vi "Test Test Fail if More than One Of.vi"(8 "error in (no error)":errorcluster, 11 "Test Case In":refnum<class "One Expectation Test.lvclass">) -> (0 "error out":errorcluster, 3 "Test Case Out":refnum<class "One Expectation Test.lvclass">)   [LabVIEW 2020, in "One Expectation Test.lvclass"]
uses:
  One Expectation Test.lvclass
  C:/Program Files (x86)/National Instruments/LabVIEW 2020/vi.lib/Astemes/LUnit/Test Case.lvclass
  <vilib>/Astemes/LUnit/Test Case.lvclass/Test Case.ctl
  <vilib>/Astemes/LUnit/Append Pass Result.vi
  <vilib>/Astemes/LUnit/Append Fail Result.vi
  <vilib>/Astemes/LUnit/Describe Comparison.vi
  <vilib>/Astemes/LUnit/Compare Variants.vi
  <vilib>/Astemes/LUnit/Variant to string.vi
  Test Interface Mock/Test Interface Mock.lvclass
  C:/git/astemes-lmock/sandbox/Mock/Mock.lvclass
  <vilib>/Utility/Data Type/Get Type Information.vi
  <vilib>/Utility/LVClass/Get LV Class Name.vi
  One Expectation Test.lvclass/One Expectation Test.ctl
  One Of/One.lvclass
  C:/git/astemes-lmock/sandbox/Test Interface Mock/Test Interface Mock.lvclass
  C:/git/astemes-lmock/sandbox/Test Interface/Test Interface.lvclass
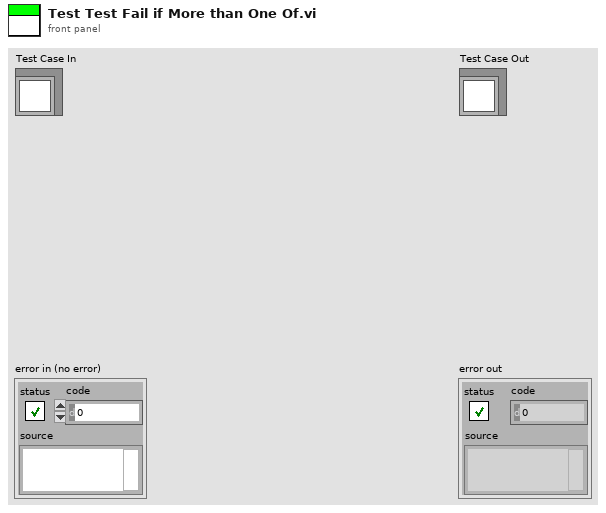
[diagram p1: front panel]
types:
  T1 = enum16{"", "Passed", "Failed", "Error", "Skipped", "Setup Error", "Broken", "Teardown Error"}
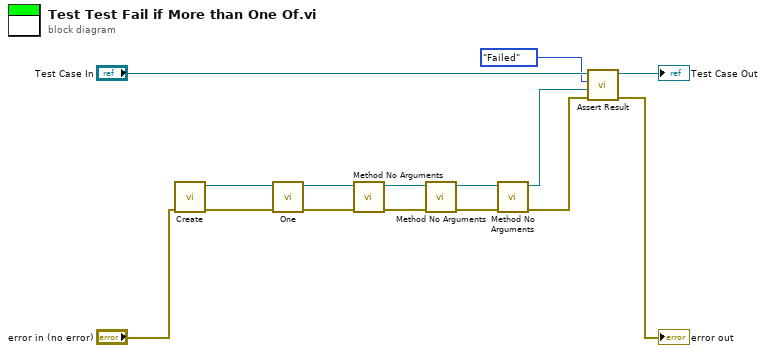
[diagram p0: block diagram]
diagram:
  n1 = call "Create.vi"("error in (no error)"="error in (no error)") -> ("error out"=w14:errorcluster, "Test Interface Mock Out"=w15:refnum<class "Test Interface Mock.lvclass">)  [unwired: 9 in]
  n2 = call "One.vi"("error in (no error)"=w14, "Mock in"=w15) -> ("error out"=w12:errorcluster, "Mock out"=w13:refnum<class "Test Interface Mock.lvclass">)  [unwired: 8 in]
  n3 = call-dynamic "Method No Arguments.vi"("error in (no error)"=w12, "Mock In"=w13) -> ("error out"=w11:errorcluster, "Mock Out"=w3:refnum<class "Test Interface Mock.lvclass">)  [unwired: 8 in]
  n4 = call-dynamic "Method No Arguments.vi"("error in (no error)"=w11, "Mock In"=w3) -> ("error out"=w4:errorcluster, "Mock Out"=w2:refnum<class "Test Interface Mock.lvclass">)  [unwired: 8 in]
  n5 = call-dynamic "Method No Arguments.vi"("error in (no error)"=w4, "Mock In"=w2) -> ("error out"=w5:errorcluster, "Mock Out"=w1:refnum<class "Test Interface Mock.lvclass">)  [unwired: 8 in]
  n6 = call "Assert Result.vi"("error in (no error)"=w5, "Mock"=w1, "Status"=T1."Failed", "One Expectation Test In"="Test Case In") -> ("error out"=→"error out":errorcluster, "One Expectation Test Out"=→"Test Case Out":refnum<class "One Expectation Test.lvclass">)  [unwired: 6 in]
